vi "Gui_SetupSequence.vi"(7 "Variant For Path":variant, 8 "error in (no error)":errorcluster, 10 "Excit Table Variant":variant, 11 "Variant":variant) -> (0 "error out":errorcluster caption="sortie d'erreur", 2 "Excit Table Variant Output":variant, 3 "Variant Output":variant)   [LabVIEW 2024]
uses:
  controls/DATA_Inputs.ctl
  controls/PROCESSING_Inputs.ctl
  controls/TRAPPING_Inputs.ctl
  controls/SEQUENCE_Inputs.ctl
  controls/EXCIT_Inputs.ctl
  controls/TIMING_Inputs.ctl
  controls/RF_TRAPPING_Inputs.ctl
panel:
  in  "Change RF Trapping":bool
  out "RF_TRAPPING Inputs":T1={"Init Values"=[0.0, 1.0, 1.0, 0.0], "Opening Values"=[0.0, -4.0, 1.0, 0.0], "Trapping Values"=[0.0, 1.0, 1.0, 0.0], "Emptying Values"=[0.0, 1.0, -7.0, 0.0], "RF Trap ON"=FALSE, "RF Accums"=1, "Number of Voltages"=4} {"RF Accums" min=1 max=100; "Trapping Values" min=-10.0 max=10.0; "Init Values" min=-10.0 max=10.0; "Emptying Values" min=-10.0 max=10.0; "Opening Values" min=-10.0 max=10.0}
  in  "SEQUENCE Inputs":T2={"EXCIT Inputs"={"Number of Excitations"=1, "Script Text"="", "Table of Waveforms"=[]}, "DATA Inputs"={"Record Length"=524000, "Sample Rate"=2000000.0, "Data Type"=0, "Vertical Range"=10.0, "Acquisition Duration"=262.0}, "TIMING Inputs"={"Number of Acquisitions "=1, "Number of Accumulations"=1, "Table of Waveforms"=[], "Script Text"=""}, "PROCESSING Inputs"={"Reference Mass"=300.0939, "Cyclotron Freq"=255.727, "Magnetron Freq"=0.001}, "TRAPPING Inputs"={"Number of Channels"=4, "Init Values"=[2.0, 9.0, 2.0, 9.0], "Opening Values"=[0.0, 0.0, 0.0, 0.0], "Trapping Values"=[2.0, 9.0, 2.0, 9.0], "Emptying Values"=[-10.0, -10.0, -10.0, -10.0], "Adiabatic ON"=FALSE, "Adiabatic Duration"=100, "Adiabatic Waveforms"=["Adiabatic_None_2_2_2000", "Adiabatic_Ramp_9_0_2000", "Adiabatic_None_2_2_2000", "Adiabatic_RC_9_0_2000"], "Ions Refill ON"=FALSE, "Number of Ions Refills"=1}, "RF_TRAPPING Inputs"={"Init Values"=[0.0, 1.0, 1.0, 0.0], "Opening Values"=[0.0, -4.0, 1.0, 0.0], "Trapping Values"=[0.0, 1.0, 1.0, 0.0], "Emptying Values"=[0.0, 1.0, -7.0, 0.0], "RF Trap ON"=FALSE, "RF Accums"=1, "Number of Voltages"=4}} {"RF_TRAPPING Inputs"."RF Accums" min=1 max=100; "RF_TRAPPING Inputs"."Trapping Values" min=-10.0 max=10.0; "RF_TRAPPING Inputs"."Init Values" min=-10.0 max=10.0; "RF_TRAPPING Inputs"."Emptying Values" min=-10.0 max=10.0; "RF_TRAPPING Inputs"."Opening Values" min=-10.0 max=10.0; "TRAPPING Inputs"."Number of Ions Refills" min=1 max=1000; "TRAPPING Inputs"."Trapping Values" min=-10.0 max=10.0; "TRAPPING Inputs"."Init Values" min=-10.0 max=10.0; "TRAPPING Inputs"."Emptying Values" min=-10.0 max=10.0; "TRAPPING Inputs"."Opening Values" min=-10.0 max=10.0; "PROCESSING Inputs"."Magnetron Freq" format="%.5g"; "PROCESSING Inputs"."Cyclotron Freq" format="%.5g"; "PROCESSING Inputs"."Reference Mass" format="%.5g"; "TIMING Inputs"."Number of Accumulations" min=0 max=50 step=1; "TIMING Inputs"."Number of Acquisitions" min=1 max=10 step=1; "DATA Inputs"."Vertical Range" items=["0.2"=0.2, "0.4"=0.4, "1"=1.0, "2"=2.0, "4"=4.0, "10"=10.0]; "DATA Inputs"."Data Type" items=["I16", "DBL"]; "DATA Inputs"."Sample Rate" items=["1 MHz"=1000000.0, "2 MHz"=2000000.0, "5 MHz"=5000000.0, "10 MHz"=10000000.0, "20 MHz"=20000000.0, "25 MHz"=25000000.0, "50 MHz"=50000000.0, "100 MHz"=100000000.0]; "EXCIT Inputs"."Number of Excitations" min=1 max=10}
  out "TRAPPING Inputs":T7={"Number of Channels"=4, "Init Values"=[2.0, 9.0, 2.0, 9.0], "Opening Values"=[0.0, 0.0, 0.0, 0.0], "Trapping Values"=[2.0, 9.0, 2.0, 9.0], "Emptying Values"=[-10.0, -10.0, -10.0, -10.0], "Adiabatic ON"=FALSE, "Adiabatic Duration"=100, "Adiabatic Waveforms"=["Adiabatic_None_2_2_2000", "Adiabatic_Ramp_9_0_2000", "Adiabatic_None_2_2_2000", "Adiabatic_RC_9_0_2000"], "Ions Refill ON"=FALSE, "Number of Ions Refills"=1} {"Number of Ions Refills" min=1 max=1000; "Trapping Values" min=-10.0 max=10.0; "Init Values" min=-10.0 max=10.0; "Emptying Values" min=-10.0 max=10.0; "Opening Values" min=-10.0 max=10.0}
  in  "Change Processing":bool
  out "PROCESSING Inputs":T6={"Reference Mass"=300.0939, "Cyclotron Freq"=255.727, "Magnetron Freq"=0.001} caption="DATA Inputs" {"Magnetron Freq" format="%.5g"; "Cyclotron Freq" format="%.5g"; "Reference Mass" format="%.5g"}
  in  "Change Trapping":bool
  in  "Change Data":bool
  out "DATA Inputs":T4={"Record Length"=100000, "Sample Rate"=10000000.0, "Data Type"=0, "Vertical Range"=10.0, "Acquisition Duration"=100000.0} {"Vertical Range" items=["0.2"=0.2, "0.4"=0.4, "1"=1.0, "2"=2.0, "4"=4.0, "10"=10.0]; "Data Type" items=["I16", "DBL"]; "Sample Rate" items=["1 MHz"=1000000.0, "2 MHz"=2000000.0, "5 MHz"=5000000.0, "10 MHz"=10000000.0, "20 MHz"=20000000.0, "25 MHz"=25000000.0, "50 MHz"=50000000.0, "100 MHz"=100000000.0]}
  in  "Change Excitation":bool
  out "Excitation Script":string
  out "Timing Script":string
  in  "Change Timing":bool
  in  "Exit":bool
  # "RF_V1"
  # "RF_V2"
  # "RF_V3"
  # "RF_V4"
  # "RF_V1"
  # "RF_V2"
  # "RF_V3"
  # "RF_V4"
  # "GO_out (Trap_in_B)"
  # "Gout (Trap_out_B)"
  # "GI_in (Trap_in_A)"
  # "Gin (Trap_out_A)"
  # "GO_out (Trap_in_B)"
  # "Gout (Trap_out_B)"
  # "GI_in (Trap_in_A)"
  # "Gin (Trap_out_A)"
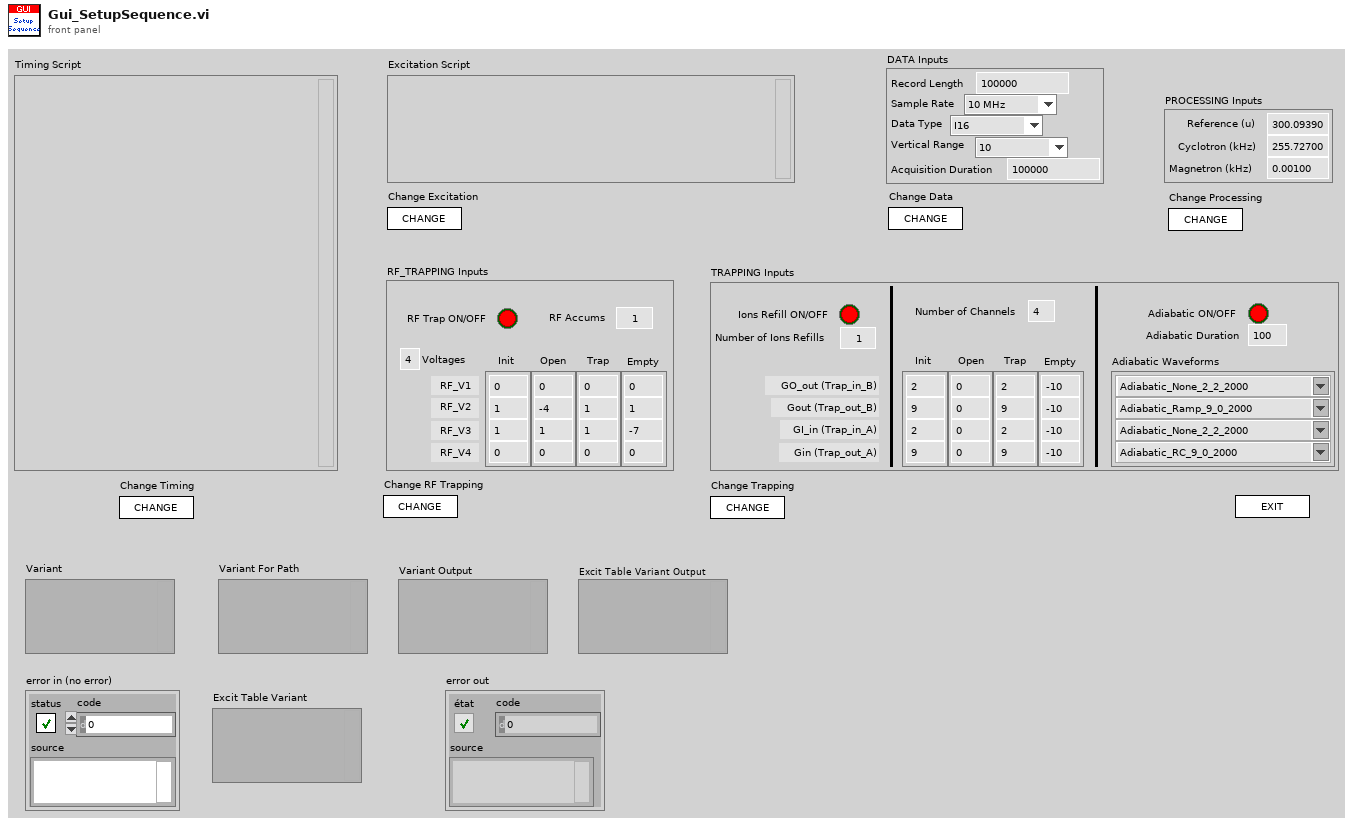
[diagram p1: front panel]
types:
  T1 = typedef "RF_TRAPPING_Inputs.ctl" = cluster{"Init Values":dbl[], "Opening Values":dbl[], "Trapping Values":dbl[], "Emptying Values":dbl[], "RF Trap ON":bool, "RF Accums":i32, "Number of Voltages":i32}
  T2 = typedef "SEQUENCE_Inputs.ctl" = cluster{"EXCIT Inputs":T3, "DATA Inputs":T4, "TIMING Inputs":T5, "PROCESSING Inputs":T6, "TRAPPING Inputs":T7, "RF_TRAPPING Inputs":T1}
  T3 = typedef "EXCIT_Inputs.ctl" = cluster{"Number of Excitations":i32, "Script Text":string, "Table of Waveforms":string[]}
  T4 = typedef "DATA_Inputs.ctl" = cluster{"Record Length":i32, "Sample Rate":dbl, "Data Type":u8, "Vertical Range":dbl, "Acquisition Duration":dbl}
  T5 = typedef "TIMING_Inputs.ctl" = cluster{"Number of Acquisitions ":i16, "Number of Accumulations":i16, "Table of Waveforms":string[], "Script Text":string}
  T6 = typedef "PROCESSING_Inputs.ctl" = cluster{"Reference Mass":dbl, "Cyclotron Freq":dbl, "Magnetron Freq":dbl}
  T7 = typedef "TRAPPING_Inputs.ctl" = cluster{"Number of Channels":i32, "Init Values":dbl[], "Opening Values":dbl[], "Trapping Values":dbl[], "Emptying Values":dbl[], "Adiabatic ON":bool, "Adiabatic Duration":i32, "Adiabatic Waveforms":string[], "Ions Refill ON":bool, "Number of Ions Refills":i32}
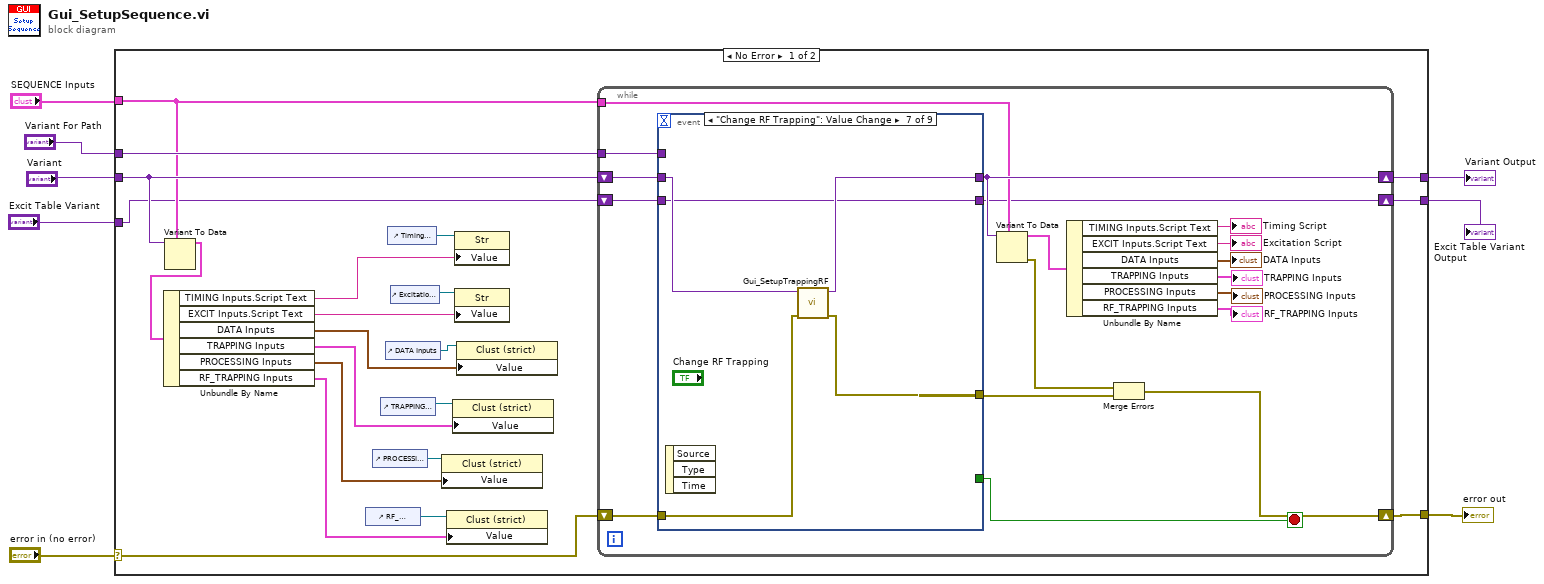
[diagram p0: block diagram]
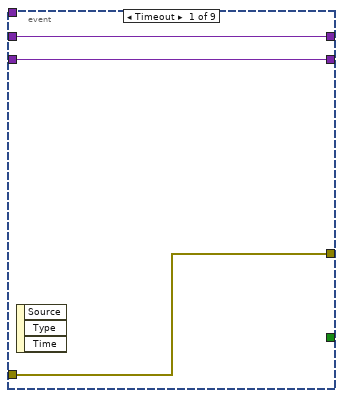
[diagram p2: hidden frame]
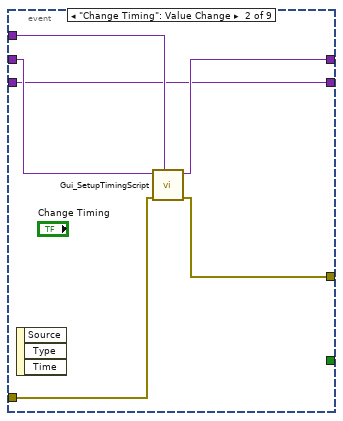
[diagram p3: hidden frame]
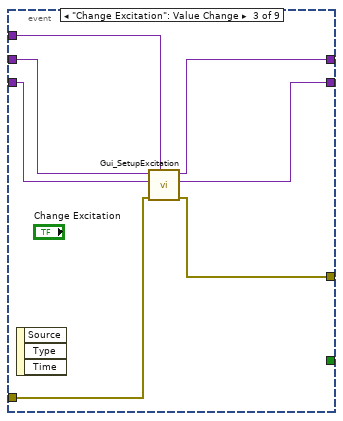
[diagram p4: hidden frame]
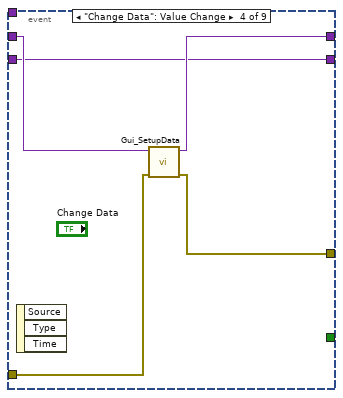
[diagram p5: hidden frame]
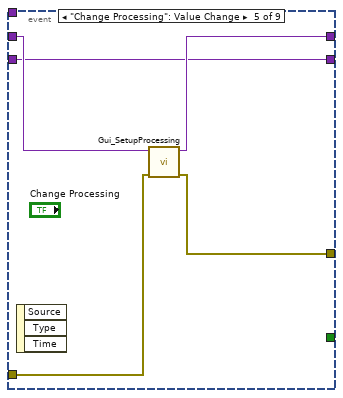
[diagram p6: hidden frame]
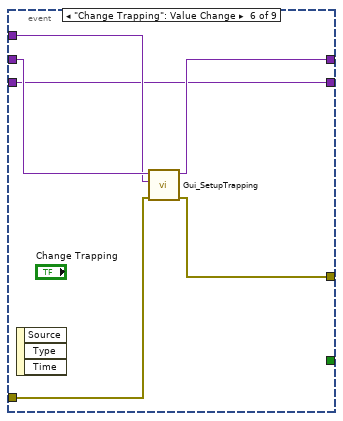
[diagram p7: hidden frame]
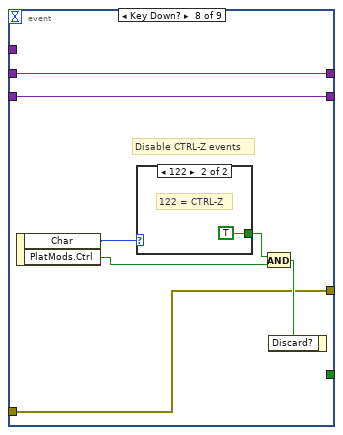
[diagram p8: hidden frame]
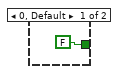
[diagram p9: hidden frame]
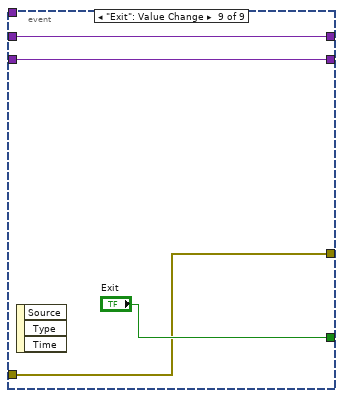
[diagram p10: hidden frame]
diagram:
  n1 = case shown="No Error" "error in (no error)" {
    selector: "error in (no error)" -> [w27 w100]
    tunnel: "Variant" -> [w25 w99]
    tunnel: [w26 w100] -> w6
    tunnel: "Variant For Path" -> [w29 _]
    tunnel: [w28 w99] -> w4
    tunnel: "SEQUENCE Inputs" -> [w17 _]
    tunnel: "Excit Table Variant" -> [w16 w98]
    tunnel: [w15 w98] -> w2
    frame No Error {
      n2 = Variant To Data(type=w17, Variant=w25) -> (data=w18:T2)  [unwired: 1 in, 1 out]
      n3 = Unbundle By Name(w18) -> ("TIMING Inputs.Script Text"=w23:string, "EXCIT Inputs.Script Text"=w21:string, "DATA Inputs"=w20:T4, "TRAPPING Inputs"=w14:T7, "PROCESSING Inputs"=w11:T6, "RF_TRAPPING Inputs"=w9:T1)
      n4 = control-ref of="RF_TRAPPING Inputs"() -> (w10:refnum<vi>)
      n5 = control-ref of="PROCESSING Inputs"() -> (w12:refnum<vi>)
      n6 = control-ref of="TRAPPING Inputs"() -> (w13:refnum<vi>)
      n7 = control-ref of="DATA Inputs"() -> (w19:refnum<vi>)
      n8 = control-ref of="Timing Script"() -> (w24:refnum<vi>)
      n9 = control-ref of="Excitation Script"() -> (w22:refnum<vi>)
      n10 = property class="Clust (strict)"(reference=w12, "Value"=w11) -> ()  [unwired: 1 in, 2 out]
      n11 = property class="Clust (strict)"(reference=w10, "Value"=w9) -> ()  [unwired: 1 in, 2 out]
      n12 = property class="Clust (strict)"(reference=w13, "Value"=w14) -> ()  [unwired: 1 in, 2 out]
      n13 = property class="Str"(reference=w24, "Value"=w23) -> ()  [unwired: 1 in, 2 out]
      n14 = property class="Str"(reference=w22, "Value"=w21) -> ()  [unwired: 1 in, 2 out]
      n15 = property class="Clust (strict)"(reference=w19, "Value"=w20) -> ()  [unwired: 1 in, 2 out]
      n16 = while {
        tunnel: w29 -> [w47]
        shift-right: [w43] -> w28
        shift-left: w25 -> [w46]
        shift-right: [w39] -> w26
        shift-left: w27 -> [w45]
        tunnel: w17 -> [w35]
        shift-right: [w33] -> w15
        shift-left: w16 -> [w32]
        stop <- w44 stop-if-true
        n17 = event shown="[6] \"Change RF Trapping\": Value Change" {
          selector: _ -> [_ _ _ _ _ _ _ _ _]
          dyn-events: _ -> [_ _ _ _ _ _ _ _ _]
          timeout: _ -> [_ _ _ _ _ _ _ _ _]
          tunnel: w47 -> [_ w55 w61 _ _ w75 _ _ _]
          tunnel: w46 -> [w49 w56 w60 w65 w70 w76 w82 w86 w96]
          tunnel: w45 -> [w50 w54 w63 w68 w73 w79 w80 w85 w95]
          tunnel: [w50 w53 w62 w66 w71 w77 w83 w85 w95] -> w40
          tunnel: [w49 w52 w57 w67 w72 w78 w84 w86 w96] -> w43
          tunnel: [_ _ _ _ _ _ _ _ "Exit"] -> w44
          tunnel: w32 -> [w48 w51 w59 w64 w69 w74 w81 w87 w94]
          tunnel: [w48 w51 w58 w64 w69 w74 w81 w87 w94] -> w33
          event Timeout {
            n18 = event-data() -> ()  [unwired: 1 in, 3 out]
          }
          event "Change Timing": Value Change {
            n19 = event-data() -> ()  [unwired: 1 in, 3 out]
            n20 = call "Gui_SetupTimingScript.vi"("Variant For Path"=w55, "error in (no error)"=w54, "Variant"=w56) -> ("error out"=w53:errorcluster, "Variant Output"=w52:variant)  [unwired: 7 in]
          }
          event "Change Excitation": Value Change {
            n21 = event-data() -> ()  [unwired: 1 in, 3 out]
            n22 = call "Gui_SetupExcitation.vi"("Variant For Path"=w61, "error in (no error)"=w63, "Excit Table Variant"=w59, "Variant"=w60) -> ("error out"=w62:errorcluster, "Excit Table Variant Output"=w58:variant, "Variant Output"=w57:variant)  [unwired: 5 in]
          }
          event "Change Data": Value Change {
            n23 = event-data() -> ()  [unwired: 1 in, 3 out]
            n24 = call "Gui_SetupData.vi"("error in (no error)"=w68, "Variant"=w65) -> ("error out"=w66:errorcluster, "Variant out"=w67:variant)  [unwired: 8 in]
          }
          event "Change Processing": Value Change {
            n25 = event-data() -> ()  [unwired: 1 in, 3 out]
            n26 = call "Gui_SetupProcessing.vi"("error in (no error)"=w73, "Variant"=w70) -> ("error out"=w71:errorcluster, "Variant out"=w72:variant)  [unwired: 8 in]
          }
          event "Change Trapping": Value Change {
            n27 = event-data() -> ()  [unwired: 1 in, 3 out]
            n28 = call "Gui_SetupTrapping.vi"("error in (no error)"=w79, "Variant for Path"=w75, "Variant"=w76) -> ("error out"=w77:errorcluster, "Variant Output"=w78:variant)  [unwired: 7 in]
          }
          event "Change RF Trapping": Value Change {
            n29 = event-data() -> ()  [unwired: 1 in, 3 out]
            n30 = call "Gui_SetupTrappingRF.vi"("error in (no error)"=w80, "Variant"=w82) -> ("error out"=w83:errorcluster, "Variant Output"=w84:variant)  [unwired: 8 in]
          }
          event Key Down? {
            # "Disable CTRL-Z events"
            n31 = event-data() -> ("Char"=w90:i16, "PlatMods.Ctrl"=w89:bool)  [unwired: 1 in]
            n32 = case shown="122" w90 {
              tunnel: [FALSE TRUE] -> w91
              frame 0, Default {
              }
              frame 122 {
                # "122 = CTRL-Z"
              }
            }
            n33 = And(x=w91, y=w89) -> (x .and. y?=w88:bool)
            n34 = event-data("Discard?"=w88) -> ()  [unwired: 1 in, 1 out]
          }
          event "Exit": Value Change {
            n35 = event-data() -> ()  [unwired: 1 in, 3 out]
          }
        }
        n36 = Variant To Data(type=w35, Variant=w43) -> (data=w42:T2, error out=w41:errorcluster)  [unwired: 1 in]
        n37 = Unbundle By Name(w42) -> ("TIMING Inputs.Script Text"=→"Timing Script":string, "EXCIT Inputs.Script Text"=→"Excitation Script":string, "DATA Inputs"=→"DATA Inputs":T4, "TRAPPING Inputs"=→"TRAPPING Inputs":T7, "PROCESSING Inputs"=→"PROCESSING Inputs":T6, "RF_TRAPPING Inputs"=→"RF_TRAPPING Inputs":T1)
        n38 = Merge Errors(w41, w40) -> (w39:errorcluster)
      }
    }
    frame Error {
    }
  }
  "error out" <- w6
  "Variant Output" <- w4
  "Excit Table Variant Output" <- w2
